vi "Main.vi"() -> ()   [LabVIEW 2013]
uses:
  <vilib>/myRIO/Common/Instrument Driver Framework/myRIO v1.0/PWM/vis/myRIO v1.1 Open PWM.vi
  <vilib>/myRIO/Common/Instrument Driver Framework/myRIO v1.0/UART/vis/myRIO v1.0 Close UART.vi
  <vilib>/myRIO/Common/Instrument Driver Framework/Utilities/vis/Validate Channels.vi
  <vilib>/myRIO/Common/Instrument Driver Framework/myRIO v1.0/PWM/vis/myRIO v1.0 Reserve PWM.vi
  <vilib>/myRIO/Common/Instrument Driver Framework/myRIO v1.0/PWM/vis/myRIO v1.0 Build MUX Configuration PWM.vi
  <vilib>/myRIO/Common/Instrument Driver Framework/myRIO v1.0/Resource Manager/vis/myRIO v1.0 Reserve Channel List.vi
  <vilib>/myRIO/Common/Instrument Driver Framework/myRIO v1.0/Resource Manager/vis/myRIO v1.0 Create Configuration List.vi
  <vilib>/myRIO/Common/Instrument Driver Framework/myRIO v1.0/Resource Manager/vis/myRIO v1.0 Reserve Channel.vi
  <vilib>/myRIO/Common/Instrument Driver Framework/myRIO v1.0/Resource Manager/vis/myRIO v1.0 Unreserve Channel.vi
  <vilib>/myRIO/Common/Instrument Driver Framework/myRIO v1.0/Resource Manager/vis/myRIO v1.0 Build Mutex Name.vi
  <vilib>/myRIO/Common/Instrument Driver Framework/myRIO v1.0/myRIO v1.1 Open.vi
  <vilib>/Utility/VariantDataType/GetNumericInfo.vi
  <vilib>/Utility/error.llb/Error Cluster From Error Code.vi
  <vilib>/myRIO/Common/Instrument Driver Framework/Utilities/vis/IO Manager.vi
  <vilib>/myRIO/Common/Instrument Driver Framework/Utilities/vis/Configuration Manager.vi
  <vilib>/myRIO/Common/Instrument Driver Framework/myRIO v1.0/Resource Manager/vis/myRIO v1.0 Configure IO.vi
  <vilib>/myRIO/Common/Instrument Driver Framework/myRIO v1.0/myRIO v1.0 Close.vi
  <vilib>/myRIO/Common/Instrument Driver Framework/myRIO v1.0/PWM/vis/myRIO v1.0 Write PWM.vi
  <vilib>/myRIO/Common/Instrument Driver Framework/Utilities/vis/FPGA Ref Manager.vi
  <vilib>/myRIO/Common/Instrument Driver Framework/myRIO v1.0/myRIO v1.0 Reset FPGA.vi
  <vilib>/myRIO/Instrument Drivers/Utilities/Utilities.lvlib
  <vilib>/myRIO/Instrument Drivers/Onboard IO/PWM/PWM.lvlib
panel:
  out "offset [%FS]":dbl
  in  "null offset":bool
  out "duty cycle [%]":dbl format="%#_3g"
  out "pulse width [ms]":dbl=1.5 format="%#_3g"
  in  "freq [Hz]":dbl=50.0
  in  "servo PWM control":tag="B/PWM0"
  out "position [%FS]":dbl(slide) scale=-200.0..200.0
  in  "[ESC]":bool
  # "Steer-by-wire demo"
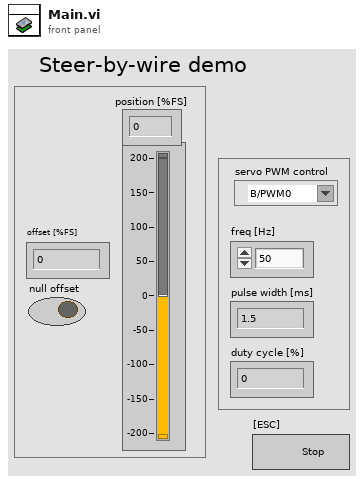
[diagram p1: front panel]
types:
  T1 = typedef "PWM.lvlib/PWM Reference.ctl" = cluster{"myRIO Reference":T2, "PWM Channels Enum":T6, "PWM Configuration":T7}
  T2 = typedef "myRIO Generic Hardware Reference.ctl" = cluster{"myRIO Model":T3, "myRIO Hardware Reference":T4}
  T3 = typedef "Hardware Version Enum.ctl" = enum16{"Unknown", "myRIO-1900", "myRIO-1950"}
  T4 = typedef "myRIO v1.0 Reference.ctl" = cluster{"Generic FPGA Reference":T5, "Allow multiple opens":bool}
  T5 = typedef "Generic FPGA Reference.ctl" = refnum<k20>
  T6 = typedef "PWM Channels Enum.ctl" = enum16{"Not Connected", "C/PWM0", "C/PWM1", "A/PWM0", "A/PWM1", "A/PWM2", "B/PWM0", "B/PWM1", "B/PWM2"}
  T7 = typedef "PWM.lvlib/PWM Configuration.ctl" = cluster{"Frequency":dbl, "Duty Cycle":dbl}
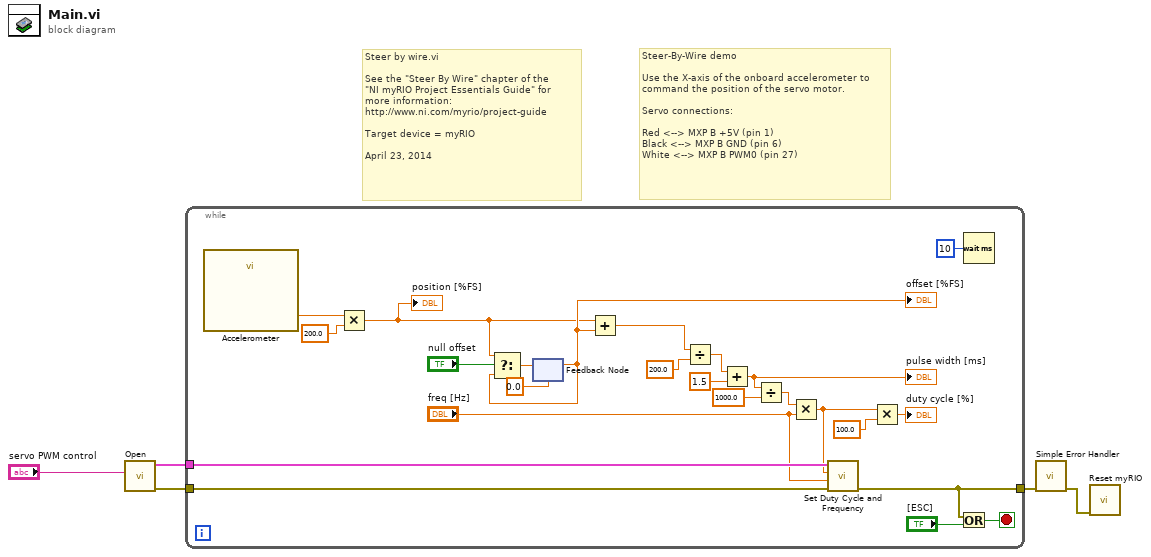
[diagram p0: block diagram]
diagram:
  # "Steer by wire.vi\n\nSee the \"Steer By Wire\" chapter of the \n\"NI myRIO Project Essentials Guide\" for\nmore information: \nhttp://www.ni.com/myrio/project-guide\n\nTarget device = myRIO\n\nApril 23, 2014"
  # "Steer-By-Wire demo\n\nUse the X-axis of the onboard accelerometer to\ncommand the position of the servo motor.\n\nServo connections:\n\nRed <--> MXP B +5V (pin 1)\nBlack <--> MXP B GND (pin 6)\nWhite <--> MXP B PWM0 (pin 27)"
  n1 = call <vilib>:"Open.vi"("Channel Name"="servo PWM control") -> ("error out"=w2:errorcluster, "PWM Ref Out"=w3:T1)  [unwired: 9 in]
  n2 = while {
    tunnel: w3 -> [w21]
    tunnel: w2 -> [w10]
    tunnel: [w9] -> w1
    stop <- w29 stop-if-true
    n3 = call "Accelerometer"() -> ("X-Axis"=w8:dbl)  [unwired: 26 in, 1 out]
    n4 = Multiply(x=w8, y=200.0) -> (x*y=w6:dbl)
    "position [%FS]" <- w6
    n5 = feedback #1(0.0 ("position [%FS]")) -> (w16:dbl)
    "offset [%FS]" <- w16
    n6 = Select(t=w6, s="null offset", f=w16) -> (s? t:f=w18:dbl)
    n7 = feedback-in #1(w18) -> ()
    n8 = Add(x=w6, y=w16) -> (x+y=w17:dbl)
    n9 = Divide(x=w17, y=200.0) -> (x/y=w25:dbl)
    n10 = Add(x=w25, y=1.5) -> (x+y=w23:dbl)
    "pulse width [ms]" <- w23
    n11 = Divide(x=w23, y=1000.0) -> (x/y=w15:dbl)
    n12 = Multiply(x=w15, y="freq [Hz]") -> (x*y=w12:dbl)
    n13 = call <vilib>:"Set Duty Cycle and Frequency.vi"("error in (no error)"=w10, "Frequency (Hz)"="freq [Hz]", "Duty Cycle (0-1)"=w12, "PWM Ref In"=w21) -> ("error out"=w9:errorcluster)  [unwired: 5 in, 1 out]
    n14 = Multiply(x=w12, y=100.0) -> (x*y=→"duty cycle [%]":dbl)
    n15 = Or(x=w9, y="[ESC]") -> (x .or. y?=w29:bool)
    n16 = Wait (ms)(milliseconds to wait=u32 10) -> ()  [unwired: 1 out]
  }
  n17 = call <vilib>:"Simple Error Handler.vi"("error in (no error)"=w1) -> ("error out"=w5:errorcluster)  [unwired: 4 in, 4 out]
  n18 = call <vilib>:"Reset myRIO.vi"("error in (no error)"=w5) -> ()  [unwired: 10 in, 1 out]
